vi "CM-Layout Slot Controls.vi"(0 "SlotRefs":refnum<vi>[](array[refnum]), 11 "error in (no error)":errorcluster) -> (15 "error out":errorcluster)   [LabVIEW 2020]
uses:
  Type Defs/General PXISlot XControl/PXISlotGP.xctl
  Type Defs/PXISlot XControl/Connector Type.ctl
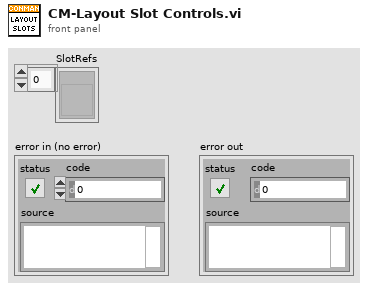
[diagram p1: front panel]
types:
  T1 = typedef "Connector Type.ctl" = enum16{"None", "PXI-4461", "BNC-2110", "BNC-2090", "PXIe-4463", "PXIe-4464"}
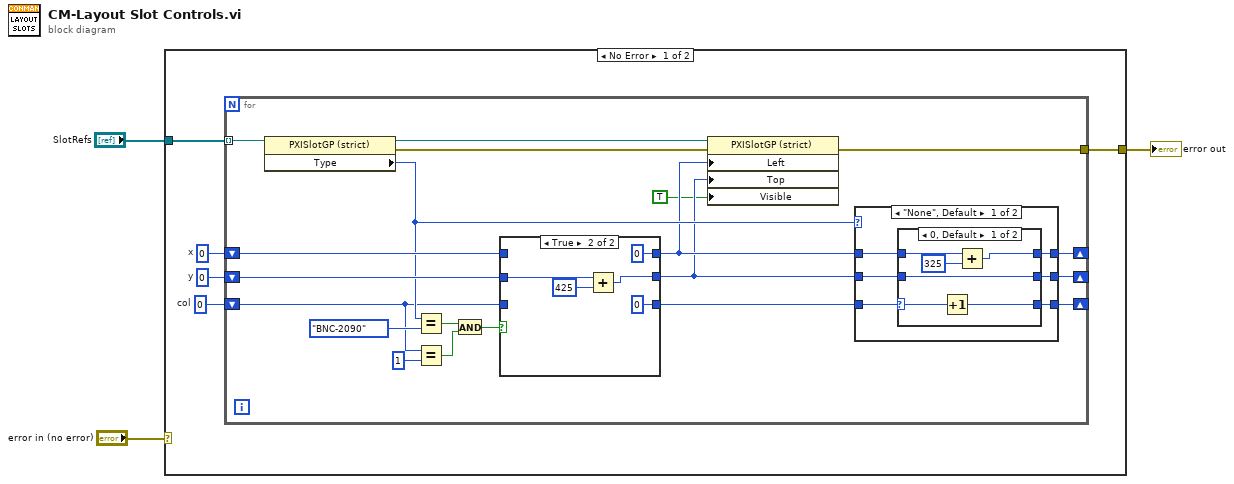
[diagram p0: block diagram]
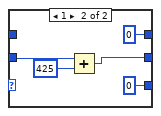
[diagram p3: hidden frame]
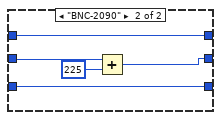
[diagram p4: hidden frame]
diagram:
  n1 = case shown="No Error" "error in (no error)" {
    selector: "error in (no error)" -> [_ w59]
    tunnel: [w4 w59] -> w2
    tunnel: "SlotRefs" -> [w6 _]
    frame No Error {
      w5 = 0  # col
      w7 = 0  # y
      w8 = 0  # x
      n2 = for {
        shift-right: [w26] -> _
        shift-left: w8 -> [w22]
        shift-right: [w27] -> _
        shift-left: w7 -> [w21]
        tunnel: w6 -> [w25] mode=indexing
        shift-right: [w28] -> _
        shift-left: w5 -> [w16]
        tunnel: [w10] -> w4
        n3 = property class="PXISlotGP (strict)"(reference=w25) -> (reference out=w24:refnum<vi>, error out=w23:errorcluster, "Type"=w20:T1)  [unwired: 1 in]
        n4 = Equal?(x=w20, y=Connector_Type."BNC-2090") -> (x = y?=w18:bool)
        n5 = Equal?(x=w16, y=1) -> (x = y?=w14:bool)
        n6 = And(x=w18, y=w14) -> (x .and. y?=w17:bool)
        n7 = case shown="True" w17 {
          tunnel: w22 -> [w31 _]
          tunnel: w21 -> [w30 w34]
          tunnel: w16 -> [w29 _]
          tunnel: [w31 0 ("x")] -> w13
          tunnel: [w30 w32] -> w12
          tunnel: [w29 0 ("col")] -> w11
          frame False {
          }
          frame True {
            n8 = Add(x=w34, y=425) -> (x+y=w32:i32)
          }
        }
        n9 = property class="PXISlotGP (strict)"(reference=w24, error in=w23, "Left"=w13, "Top"=w12, "Visible"=TRUE) -> (error out=w10:errorcluster)  [unwired: 1 out]
        n10 = case shown="\"None\", Default" w20 {
          tunnel: w13 -> [w38 w57]
          tunnel: w12 -> [w40 w56]
          tunnel: w11 -> [w42 w58]
          tunnel: [w41 w58] -> w28
          tunnel: [w39 w54] -> w27
          tunnel: [w37 w57] -> w26
          frame "None", Default {
            n11 = case shown="0, Default" w42 {
              selector: w42 -> [w48 _]
              tunnel: [w47 0] -> w41
              tunnel: w40 -> [w46 w51]
              tunnel: [w46 w49] -> w39
              tunnel: w38 -> [w45 _]
              tunnel: [w43 0] -> w37
              frame 0, Default {
                n12 = Increment(x=w48) -> (x+1=w47:i32)
                n13 = Add(x=w45, y=325) -> (x+y=w43:i32)
              }
              frame 1 {
                n14 = Add(x=w51, y=425) -> (x+y=w49:i32)
              }
            }
          }
          frame "BNC-2090" {
            n15 = Add(x=w56, y=225) -> (x+y=w54:i32)
          }
        }
      }
    }
    frame Error {
    }
  }
  "error out" <- w2
